vi "DAQ.Sync.vi"(8 "error in (no error)":errorcluster, 11 "DAQmx in":refnum<class "DAQmx.lvclass">) -> (0 "error out":errorcluster, 3 "DAQmx out":refnum<class "DAQmx.lvclass">)   [LabVIEW 2016, in "DAQmx.lvclass"]
uses:
  DAQmx.lvclass
  DAQmx.lvclass/DAQmx.ctl
  <vilib>/DAQmx/configure/trigger.llb/DAQmx Start Trigger (Digital Edge).vi
  <resource>/objmgr/daqmx.rc
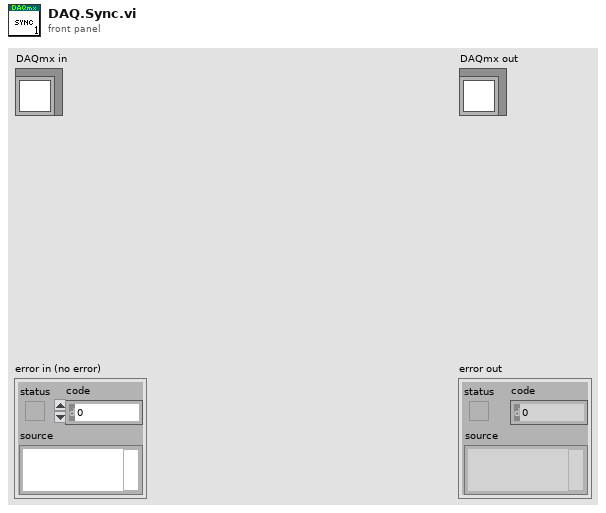
[diagram p1: front panel]
types:
  T1 = cluster{"RefClk.Src":tag, "SyncPulse.src":tag, "StartTrigger.src":tag, "SyncPulse.SyncTime":dbl}
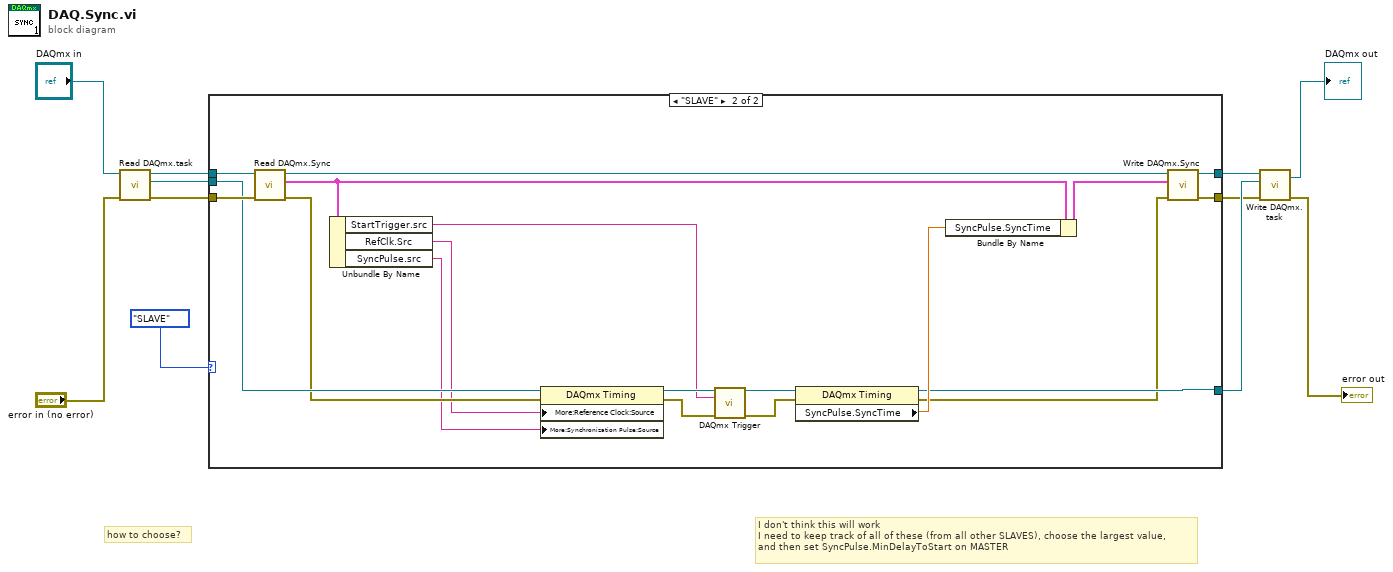
[diagram p0: block diagram]
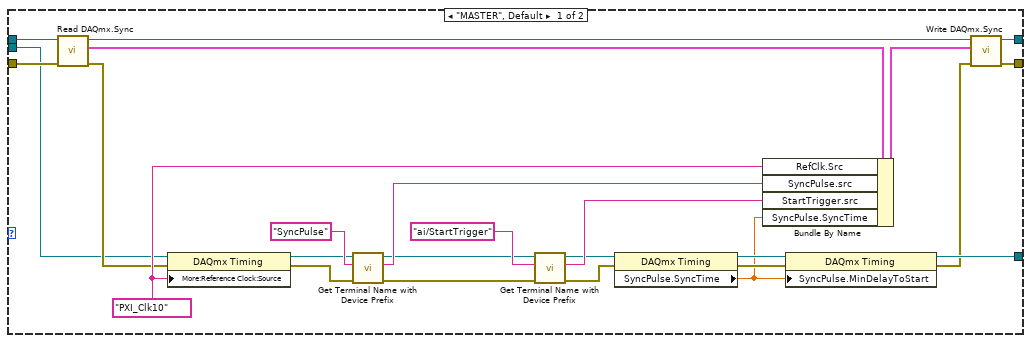
[diagram p2: hidden frame]
diagram:
  # "I don't think this will work\nI need to keep track of all of these (from all other SLAVES), choose the largest value,\nand then set SyncPulse.MinDelayToStart on MASTER"
  # "how to choose?"
  n1 = call "Read DAQmx.task.vi"("error in (no error)"="error in (no error)", "DAQmx in"="DAQmx in") -> ("error out"=w3:errorcluster, "task"=w7:refnum<k21>, "DAQmx out"=w5:refnum<class "DAQmx.lvclass">)  [unwired: 7 in]
  n2 = case shown="\"SLAVE\"" enum16{"MASTER", "SLAVE"}."SLAVE" {
    tunnel: w7 -> [w17 w51]
    tunnel: [w14 w38] -> w6
    tunnel: w3 -> [w22 w52]
    tunnel: w5 -> [w25 w55]
    tunnel: [w23 w54] -> w4
    tunnel: [w18 w41] -> w2
    frame "MASTER", Default {
      w27 = tag "PXI_Clk10" ("RefClk.Src")
      n3 = call "Read DAQmx.Sync.vi"("error in (no error)"=w22, "DAQmx in"=w25) -> ("error out"=w21:errorcluster, "Sync"=w20:T1, "DAQmx out"=w24:refnum<class "DAQmx.lvclass">)  [unwired: 7 in]
      n4 = property class="DAQmx Timing"(reference=w17, error in=w21, "More:Reference Clock:Source"=w27) -> (reference out=w34:refnum<k21>, error out=w33:errorcluster)
      n5 = call "Get Terminal Name with Device Prefix.vi"("error in (no error)"=w33, "Local Terminal Name"="SyncPulse", "task/channels in"=w34) -> ("error out"=w30:errorcluster, "Terminal Name with Device Prefix"=w32:tag, "task out"=w31:refnum<k21>)  [unwired: 6 in]
      n6 = call "Get Terminal Name with Device Prefix.vi"("error in (no error)"=w30, "Local Terminal Name"="ai/StartTrigger", "task/channels in"=w31) -> ("error out"=w26:errorcluster, "Terminal Name with Device Prefix"=w29:tag, "task out"=w28:refnum<k21>)  [unwired: 6 in]
      n7 = property class="DAQmx Timing"(reference=w28, error in=w26) -> (reference out=w16:refnum<k21>, error out=w15:errorcluster, "SyncPulse.SyncTime"=w12:dbl)
      n8 = Bundle By Name(cluster=w20, "RefClk.Src"=w27, "SyncPulse.src"=w32, "StartTrigger.src"=w29, "SyncPulse.SyncTime"=w12) -> (w19:T1)
      n9 = property class="DAQmx Timing"(reference=w16, error in=w15, "SyncPulse.MinDelayToStart"=w12) -> (reference out=w14:refnum<k21>, error out=w13:errorcluster)
      n10 = call "Write DAQmx.Sync.vi"("error in (no error)"=w13, "Sync"=w19, "DAQmx in"=w24) -> ("error out"=w18:errorcluster, "DAQmx out"=w23:refnum<class "DAQmx.lvclass">)  [unwired: 7 in]
    }
    frame "SLAVE" {
      n11 = call "Read DAQmx.Sync.vi"("error in (no error)"=w52, "DAQmx in"=w55) -> ("error out"=w50:errorcluster, "Sync"=w42:T1, "DAQmx out"=w53:refnum<class "DAQmx.lvclass">)  [unwired: 7 in]
      n12 = Unbundle By Name(w42) -> ("StartTrigger.src"=w40:tag, "RefClk.Src"=w45:tag, "SyncPulse.src"=w44:tag)
      n13 = property class="DAQmx Timing"(reference=w51, error in=w50, "More:Reference Clock:Source"=w45, "More:Synchronization Pulse:Source"=w44) -> (reference out=w48:refnum<k21>, error out=w49:errorcluster)
      n14 = call-poly <vilib>:"DAQmx Trigger.vi"("task/channels in"=w48, "source"=w40, "error in"=w49) -> ("task out"=w47:refnum<k21>, "error out"=w46:errorcluster)  [unwired: 11 in]
      n15 = property class="DAQmx Timing"(reference=w47, error in=w46) -> (reference out=w38:refnum<k21>, error out=w37:errorcluster, "SyncPulse.SyncTime"=w39:dbl)
      n16 = Bundle By Name(cluster=w42, "SyncPulse.SyncTime"=w39) -> (w43:T1)
      n17 = call "Write DAQmx.Sync.vi"("error in (no error)"=w37, "Sync"=w43, "DAQmx in"=w53) -> ("error out"=w41:errorcluster, "DAQmx out"=w54:refnum<class "DAQmx.lvclass">)  [unwired: 7 in]
    }
  }
  n18 = call "Write DAQmx.task.vi"("error in (no error)"=w2, "task"=w6, "DAQmx in"=w4) -> ("error out"=→"error out":errorcluster, "DAQmx out"=→"DAQmx out":refnum<class "DAQmx.lvclass">)  [unwired: 7 in]
